vi "Voltage to Distance2.vi"(0 "Voltage":dbl, 1 "Calibration Parameters":cluster{"a":dbl, "b":dbl, "c":dbl, "d":dbl}={"a"=4.76809, "b"=2.19854, "c"=3.45456, "d"=0.0655}) -> (7 "Distance":dbl)   [LabVIEW 2016]
doc: "Convert the raw data of voltages to distance values in meter.\n\nUse the Calibration VI to calculate the calibration parameters."
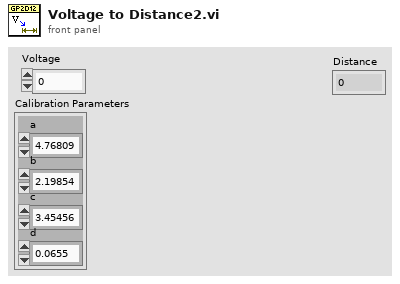
[diagram p1: front panel]
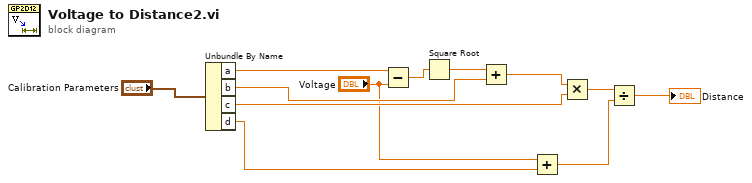
[diagram p0: block diagram]
diagram:
  n1 = Unbundle By Name("Calibration Parameters") -> ("a"=w11:dbl, "b"=w8:dbl, "c"=w6:dbl, "d"=w1:dbl)
  n2 = Subtract(x=w11, y="Voltage") -> (x-y=w10:dbl)
  n3 = Square Root(x=w10) -> (sqrt(x)=w9:dbl)
  n4 = Add(x=w9, y=w8) -> (x+y=w7:dbl)
  n5 = Add(x="Voltage", y=w1) -> (x+y=w3:dbl)
  n6 = Multiply(x=w7, y=w6) -> (x*y=w4:dbl)
  n7 = Divide(x=w4, y=w3) -> (x/y=→"Distance":dbl)
